vi "get_ROI_intensity_series.vi"(8 "error in (no error)":errorcluster, 10 "ROIs":T1(array[cluster]) {"Contours"."Type" items=["No Selection", "Point", "Line", "Rectangle", "Oval", "Polygon", "Freehand Region", "Annulus", "Unused2", "Unused3", "Broken Line", "Freehand Line", "Rotated Rectangle"]}, 11 "ImageCollection in":refnum<class "ImageCollection.lvclass">) -> (0 "error out":errorcluster, 2 "intensity series":dbl[][](array[numeric]), 3 "ImageCollection out":refnum<class "ImageCollection.lvclass">)   [LabVIEW 2010, in "ImageCollection.lvclass"]
uses:
  ImageCollection.lvclass
  Image/Image/Image.lvclass
  Image/Image/storage_mode.ctl
  ImageCollection.lvclass/ImageCollection.ctl
  <vilib>/vision/NI_Vision_Development_Module.lvlib
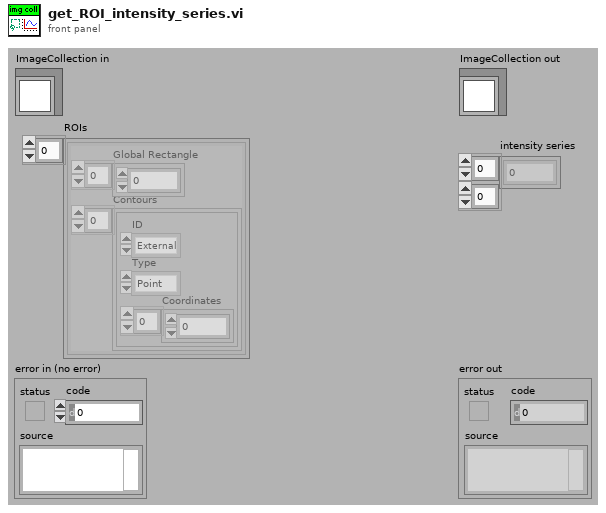
[diagram p1: front panel]
types:
  T1 = cluster{"Global Rectangle":i32[], "Contours":cluster{"ID":enum32{"External", "Internal"}, "Type":u32, "Coordinates":i32[]}[]}[]
  T2 = typedef "Image.lvclass/storage_mode.ctl" = enum16{"RAM", "disk"}
  T3 = typedef "IMAQ Image.ctl" = refnum<image>
  T4 = typedef "Image Type" = u32
  T5 = cluster{"Min":sgl, "Max":sgl, "Mean":sgl, "Std Dev":sgl, "Count":i32}
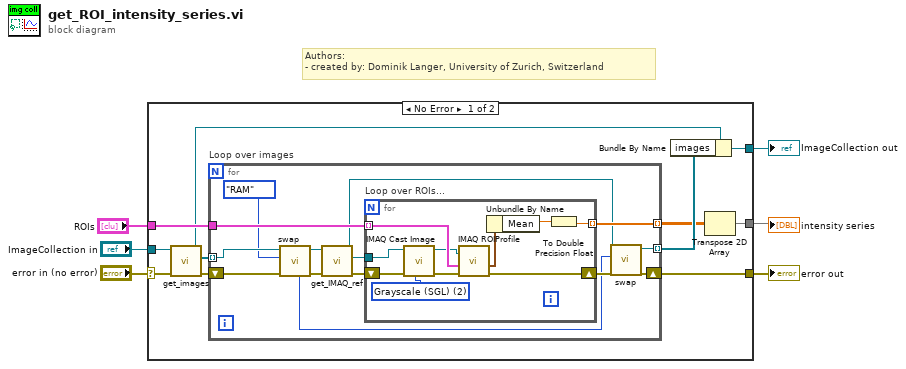
[diagram p0: block diagram]
diagram:
  # "Authors: \n- created by: Dominik Langer, University of Zurich, Switzerland"
  n1 = case shown="No Error" "error in (no error)" {
    selector: "error in (no error)" -> [w16 w43]
    tunnel: [w17 w43] -> w5
    tunnel: [w9 w42] -> w3
    tunnel: "ImageCollection in" -> [w15 w42]
    tunnel: "ROIs" -> [w12 _]
    tunnel: [w8 _] -> w2
    frame No Error {
      n2 = call-dynamic "get_images.vi"("error in (no error)"=w16, "ImageCollection.lvclass in"=w15) -> ("error out"=w14:errorcluster, "images"=w13:refnum<class "Image.lvclass">[], "ImageCollection.lvclass out"=w10:refnum<class "ImageCollection.lvclass">)  [unwired: 7 in]
      n3 = for "Loop over images" {
        tunnel: w13 -> [w25] mode=indexing
        shift-right: [w21] -> w17
        shift-left: w14 -> [w27]
        tunnel: [w29] -> w7 mode=indexing
        tunnel: w12 -> [w28]
        tunnel: [w19] -> w11 mode=indexing
        n4 = call-dynamic "swap.vi"("error in (no error)"=w27, "storage type target"=storage_mode."RAM", "Image in"=w25) -> ("error out"=w26:errorcluster, "Image out"=w24:refnum<class "Image.lvclass">, "previous storage mode"=w18:T2)  [unwired: 6 in]
        n5 = call-dynamic "get_IMAQ_ref.vi"("error in (no error)"=w26, "Image.lvclass in"=w24) -> ("error out"=w31:errorcluster, "Image"=w30:T3, "Image.lvclass out"=w20:refnum<class "Image.lvclass">)  [unwired: 5 in, 2 out]
        n6 = for "Loop over ROIs..." {
          tunnel: w30 -> [w34]
          tunnel: [w37] -> w29 mode=indexing
          tunnel: w28 -> [w39] mode=indexing
          shift-right: [w41] -> w22
          shift-left: w31 -> [w36]
          w32 = T4 2 items=["Grayscale (U8)", "Grayscale (I16)", "Grayscale (SGL)", "Complex (CSG)", "RGB (U32)", "HSL (U32)", "RGB (U64)", "Grayscale (U16)"] ("Image Type")
          n7 = call "IMAQ Cast Image"("Image Type"=w32, "error in (no error)"=w36, "Image Src"=w34) -> ("error out"=w35:errorcluster, "Image Dst Out"=w33:T3)  [unwired: 7 in]
          n8 = call "IMAQ ROIProfile"("error in (no error)"=w35, "ROI Descriptor"=w39, "Image"=w33) -> ("ROI Pixel Statistics"=w40:T5, "error out"=w41:errorcluster)  [unwired: 4 out]
          n9 = Unbundle By Name(w40) -> ("Mean"=w38:sgl)
          n10 = To Double Precision Float(number=w38) -> (double precision float=w37:dbl)
        }
        n11 = call-dynamic "swap.vi"("error in (no error)"=w22, "storage type target"=w18, "Image in"=w20) -> ("error out"=w21:errorcluster, "Image out"=w19:refnum<class "Image.lvclass">)  [unwired: 6 in, 1 out]
      }
      n12 = Bundle By Name(cluster=w10, "images"=w11) -> (w9:refnum<class "ImageCollection.lvclass">)
      n13 = Transpose 2D Array(2D array=w7) -> (transposed array=w8:dbl[][])
    }
    frame Error {
    }
  }
  "error out" <- w5
  "ImageCollection out" <- w3
  "intensity series" <- w2
